vi "load cvt1 taglist.vi"(9 "target name":string, 10 "cfg file path":path, 11 "vi path":path) -> (2 "ok?":bool, 3 "tags":refnum<class "tag descriptor.lvclass">[](array[class]))   [LabVIEW 2013, in "PL Framework Configuration Tool.lvlib" / "EngineTags.lvclass"]
uses:
  EngineTags.lvclass
  <vilib>/NI/Tag Bus/tag/tag descriptor.lvclass
  <vilib>/NI/Tag Bus/tag/Data Type.ctl
  <vilib>/NI/Tag Bus/tag/tag descriptor.lvclass/tag descriptor.ctl
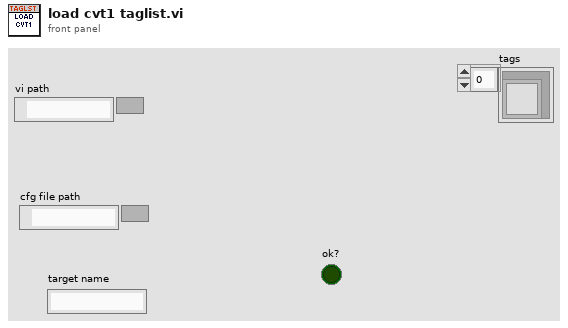
[diagram p1: front panel]
types:
  T1 = cluster{"Name":string, "Data Type":enum16{"Bool", "U8", "I32", "Double", "String", "Enum"}, "Array":bool, "Size":u32, "Default":string, "Enum":string[], "Description":string}[]
  T2 = typedef "tag bus.lvlib/tag descriptor.lvclass/Data Type.ctl" = enum16{"Double", "Single", "I64", "I32", "I16", "I8", "U64", "U32", "U16", "U8", "Boolean", "String", "Array of Double", "Array of Single", "Array of I64", "Array of I32", "Array of I16", "Array of I8", "Array of U64", "Array of U32", "Array of U16", "Array of U8", "Array of Boolean", "Array of String"}
  T3 = enum16{"Bool", "U8", "I32", "Double", "String", "Enum"}
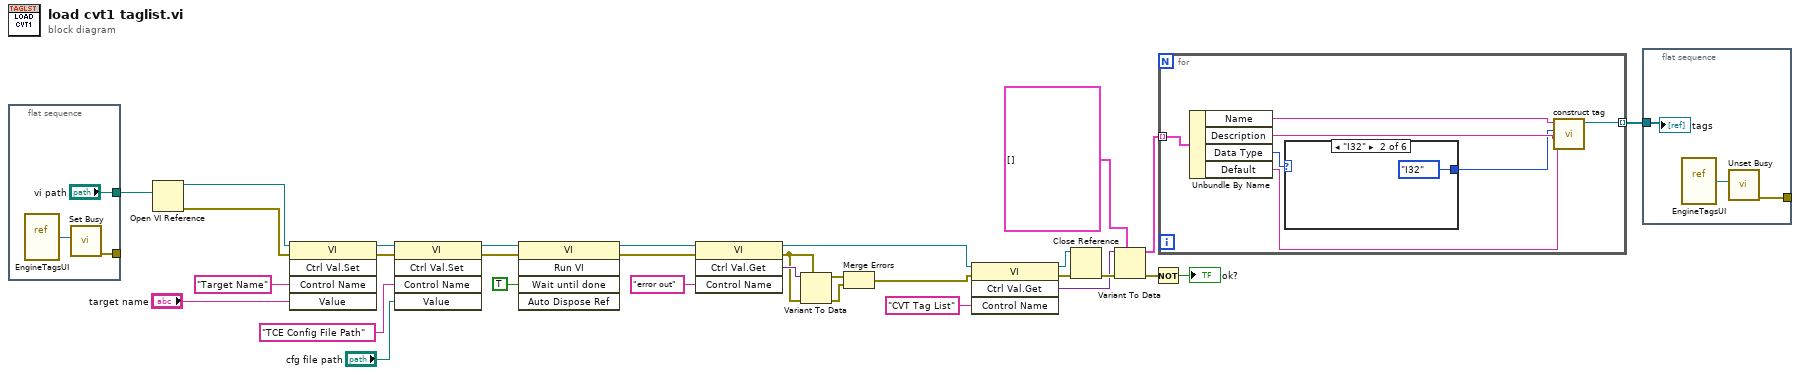
[diagram p0: block diagram]
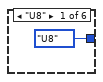
[diagram p2: hidden frame]
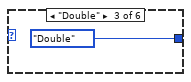
[diagram p3: hidden frame]
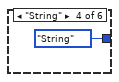
[diagram p4: hidden frame]
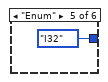
[diagram p5: hidden frame]
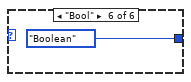
[diagram p6: hidden frame]
diagram:
  n1 = flat-sequence {
    tunnel: [w33] -> _
    tunnel: ["vi path"] -> w2
    frame #0 {
      n2 = vi-ref "EngineTagsUI.vi"() -> (w34:refnum<vi>)
      n3 = call <vilib>:"Set Busy.vi"("VI reference (current VI)"=w34) -> ("error out"=w33:errorcluster)  [unwired: 9 in, 1 out]
    }
  }
  n4 = Open VI Reference(vi path=w2) -> (vi reference=w30:refnum<vi>, error out=w31:errorcluster)  [unwired: 5 in]
  n5 = invoke class="VI" method="Ctrl Val.Set"(reference=w30, error in=w31, "Control Name"="Target Name", "Value"="target name") -> (reference out=w28:refnum<vi>, error out=w29:errorcluster)  [unwired: 1 in, 3 out]
  n6 = invoke class="VI" method="Ctrl Val.Set"(reference=w28, error in=w29, "Control Name"="TCE Config File Path", "Value"="cfg file path") -> (reference out=w5:refnum<vi>, error out=w26:errorcluster)  [unwired: 1 in, 3 out]
  n7 = invoke class="VI" method="Run VI"(reference=w5, error in=w26, "Wait until done"=TRUE ("Wait Until Done")) -> (reference out=w4:refnum<vi>, error out=w6:errorcluster)  [unwired: 2 in, 3 out]
  n8 = invoke class="VI" method="Ctrl Val.Get"(reference=w4, error in=w6, "Control Name"="error out") -> (reference out=w27:refnum<vi>, error out=w18:errorcluster, "Get Control Value Variant"=w19:variant)  [unwired: 1 in, 1 out]
  n9 = Variant To Data(error in=w18, type=w18, Variant=w19) -> (data=w16:errorcluster, error out=w20:errorcluster)
  n10 = Merge Errors(w16, w20) -> (w17:errorcluster)
  n11 = invoke class="VI" method="Ctrl Val.Get"(reference=w27, error in=w17, "Control Name"="CVT Tag List") -> (reference out=w12:refnum<vi>, error out=w14:errorcluster, "Get Control Value Variant"=w9:variant)  [unwired: 1 in, 1 out]
  n12 = Close Reference(reference=w12, error in (no error)=w14) -> (error out=w13:errorcluster)
  n13 = Variant To Data(error in=w13, type=T1 [], Variant=w9) -> (data=w7:T1, error out=w11:errorcluster)
  n14 = Not(x=w11) -> (.not. x?=→"ok?":bool)
  n15 = for {
    tunnel: w7 -> [w41] mode=indexing
    tunnel: [w36] -> w1 mode=indexing
    n16 = Unbundle By Name(w41) -> ("Name"=w39:string, "Description"=w38:string, "Data Type"=w40:T3, "Default"=w35:string)
    n17 = case shown="\"I32\"" w40 {
      tunnel: [Data_Type."U8" ("Data Type") Data_Type."I32" ("Data Type") Data_Type."Double" ("Data Type") Data_Type."String" ("Data Type") Data_Type."I32" ("Data Type") Data_Type."Boolean" ("Data Type")] -> w37
      frame "U8" {
      }
      frame "I32" {
      }
      frame "Double" {
      }
      frame "String" {
      }
      frame "Enum" {
      }
      frame "Bool" {
      }
    }
    n18 = call <vilib>:"construct tag.vi"("raw default"=w35, "metadata"=w38, "data type"=w37, "name"=w39) -> ("system tag out"=w36:refnum<class "tag descriptor.lvclass">)  [unwired: 7 in]
  }
  n19 = flat-sequence {
    tunnel: [w49] -> _
    tunnel: w1 -> [w48]
    frame #0 {
      n20 = vi-ref "EngineTagsUI.vi"() -> (w50:refnum<vi>)
      n21 = call <vilib>:"Unset Busy.vi"("VI reference (current VI)"=w50) -> ("error out"=w49:errorcluster)  [unwired: 10 in]
      "tags" <- w48
    }
  }
